vi "Pressure Regulator Test Interface.vi"() -> ()   [LabVIEW 2012, in "Pressure Regulator Controller.lvlib"]
uses:
  Pressure Regulator Controller.lvlib
  <vilib>/express/express shared/transition.llb/Dynamic To Waveform Array.vi
  <vilib>/express/express signal manip/GetorSetDDTAttributes/Shared VIs/XDimension conversion.vi
  <vilib>/express/express signal manip/GetorSetDDTAttributes/Get DDT Attributes/Get DDT Properties.xnode
  <vilib>/express/express signal manip/GetorSetDDTAttributes/Shared VIs/XDimension.ctl
  <vilib>/express/express signal manip/GetorSetDDTAttributes/Shared VIs/GetSetShared.lvlib
panel:
  out "Pressure":dynamicdata(graph)
  out "Signals":dynamicdata(graph)
  in  "stop (F)":bool
  out "error out":errorcluster
  in  "High Level Controls":T1={"Record Button"=FALSE, "Exit"=FALSE, "Hunt"=FALSE, "Break In"=FALSE, "Seal"=FALSE, "Drive In"=FALSE, "Load Pipette"=FALSE, "REC"=FALSE, "File Path Control"=path "D:/Rita Logfiles", "Auto Button"=FALSE, "Auto"=FALSE, "Engage Target"=FALSE, "Abort"=FALSE}
  in  "Calibration Parameters":T2={"Test Signal"={"Seal"={"Amplitude [mV]"=30, "Frequency [hz]"=100}, "Extracellular"={"Amplitude [mV]"=10, "Frequency [hz]"=100}}, "Capacitance Compensation"={"Iterations"=2, "Timeout [ms]"=3000}, "Holding Potential Dynamics"={"Start [mV]"=-70.0, "Target [mV]"=-70.0, "Speed [mV/s]"=0.0}, "Manipulator Dynamics"={"Step length [um]"=2.0, "Interstep Interval [ms]"=3000, "Initial Speed [um/s]"=10.0, "Max Speed [um/s]"=10.0, "Acceleration [um/s^2]"=10.0, "Max Depth [um]"=1200.0, "Max Penetration [um]"=1200.0}, "Suction Parameters"={"Initial Pressure [Kpa]"=0.0, "Minimum Pressure [KPa]"=-40.0, "Decremental Step [KPa]"=-2.0, "Decremental Threshold [%]"=10.0, "Falloff Threshold [%]"=5.0, "Falloff Lag [ms]"=10000.0, "Monitor Refresh [ms]"=3000.0}, "Pressure SPs [KPa]"={"High"=50.0, "Low"=15.0}, "Seal Parameters"={"Seal Target [MOhm]"=1000.0, "Stability Threhsold [%]"=10.0, "Seal Timeout [s]"=600.0, "Stability Refresh [ms]"=3000.0}, "Break in pulse Dynamics"={"Length [ms]"=200.0, "Voltage [mV]"=1000.0, "Pressure [KPa]"=-20.0}, "Unblockage Parameters"={"Blockage Threshold [%]"=5.0, "Max Attempt"=3}, "Targeter Settings"={"Approaching Calibration"={"Approach Factor [um]"=0.9, "Final Clearance [um]"=2.0}, "Optic Flow Settings"={"Pyramid Levels"=6, "Max Iterations"=8, "Displacement Threshold"=0.0, "Window Size"=45}, "Focus"={"Timeout [ms]"=5000, "Max Attempts"=2, "Method"=enum."Continuous"}}} {"Test Signal"."Extracellular"."Frequency [hz]" items=["2 hz "=2, "5 hz"=5, "10 hz "=10, "20 hz"=20, "50 hz"=50, "60 hz"=60, "100 hz"=100, "200 hz"=200, "500 hz"=500, "1000 hz"=1000]; "Test Signal"."Seal"."Frequency [hz]" items=["2 hz "=2, "5 hz"=5, "10 hz "=10, "20 hz"=20, "50 hz"=50, "60 hz"=60, "100 hz"=100, "200 hz"=200, "500 hz"=500, "1000 hz"=1000]}
  in  "Pressure Controls":T3 {"Pressure Sp Manual [KPa]" scale=-50.0..100.0}
  in  "Hardware Configuration":T4={"Pressure Controller Dynamics"={"Positive Branch"={"Kp"=0.0007, "Ki"=0.06, "Kd"=1.0}, "Negative Branch"={"Kp"=0.005, "Ki"=0.005, "Kd"=2.0}}, "Amplifier"={"Multiclamp Serial Number"="00832548", "Multiclamp Channel"=0}, "Manipulator Port"="COM10", "Objective"=600, "Sciscan core Ref"=path "C:/Users/Southampton/Desktop/LUCA_SciScan_141211/GFG/GFG_core.ref", "Signals Sampling"={"Sample Mode"=10123, "Sampling frequecy [hz]"=20000.0, "Samples Number"=1000}, "Electrode Signal"={"Scale Type"=10348, "Terminal Configuration"=10083, "Scale Name"="", "Range [V]"={"max"=10.0, "min"=-10.0}, "Physical Channel"="Dev4/ai2"}, "Pressure Signal"={"Scale Type"=10065, "Terminal Configuration"=10083, "Scale Name"="Compund Pressure", "Range [V]"={"max"=4.0, "min"=0.0}, "Physical Channel"="Dev4/ai4"}, "IIR Filter Specifications"={"Topology"=enum."Off", "Type"=enum."Lowpass", "Order"=0, "Lower Fc"=0.0, "Upper Fc"=0.0, "PB Ripple"=0.0, "SB Attenuation"=0.0}, "Pressure Controller Port"="COM8", "Scope Dynamics"={"Initial Speed [um/s]"=500.0, "Max Speed [um/s]"=1000.0, "Acceleration [um/s^2]"=25.0, "Max Depth [um]"=5000.0}} {"Pressure Signal"."Terminal Configuration" items=["Default"=-1, "RSE"=10083, "Differential"=10106, "Pseudodifferential"=12529]; "Pressure Signal"."Scale Type" items=["Volts"=10348, "Custom Scale"=10065]; "Electrode Signal"."Terminal Configuration" items=["Default"=-1, "RSE"=10083, "Differential"=10106, "Pseudodifferential"=12529]; "Electrode Signal"."Scale Type" items=["Volts"=10348, "Custom Scale"=10065]; "Signals Sampling"."Sample Mode" items=["Finite Samples"=10178, "Continuous Samples"=10123, "Hardware Timed Single Point"=12522]; "Objective" items=["Nikon 16x / 0.80w"=600]; "Amplifier"."Multiclamp Channel" items=["Channel 1", "Channel 2"]}
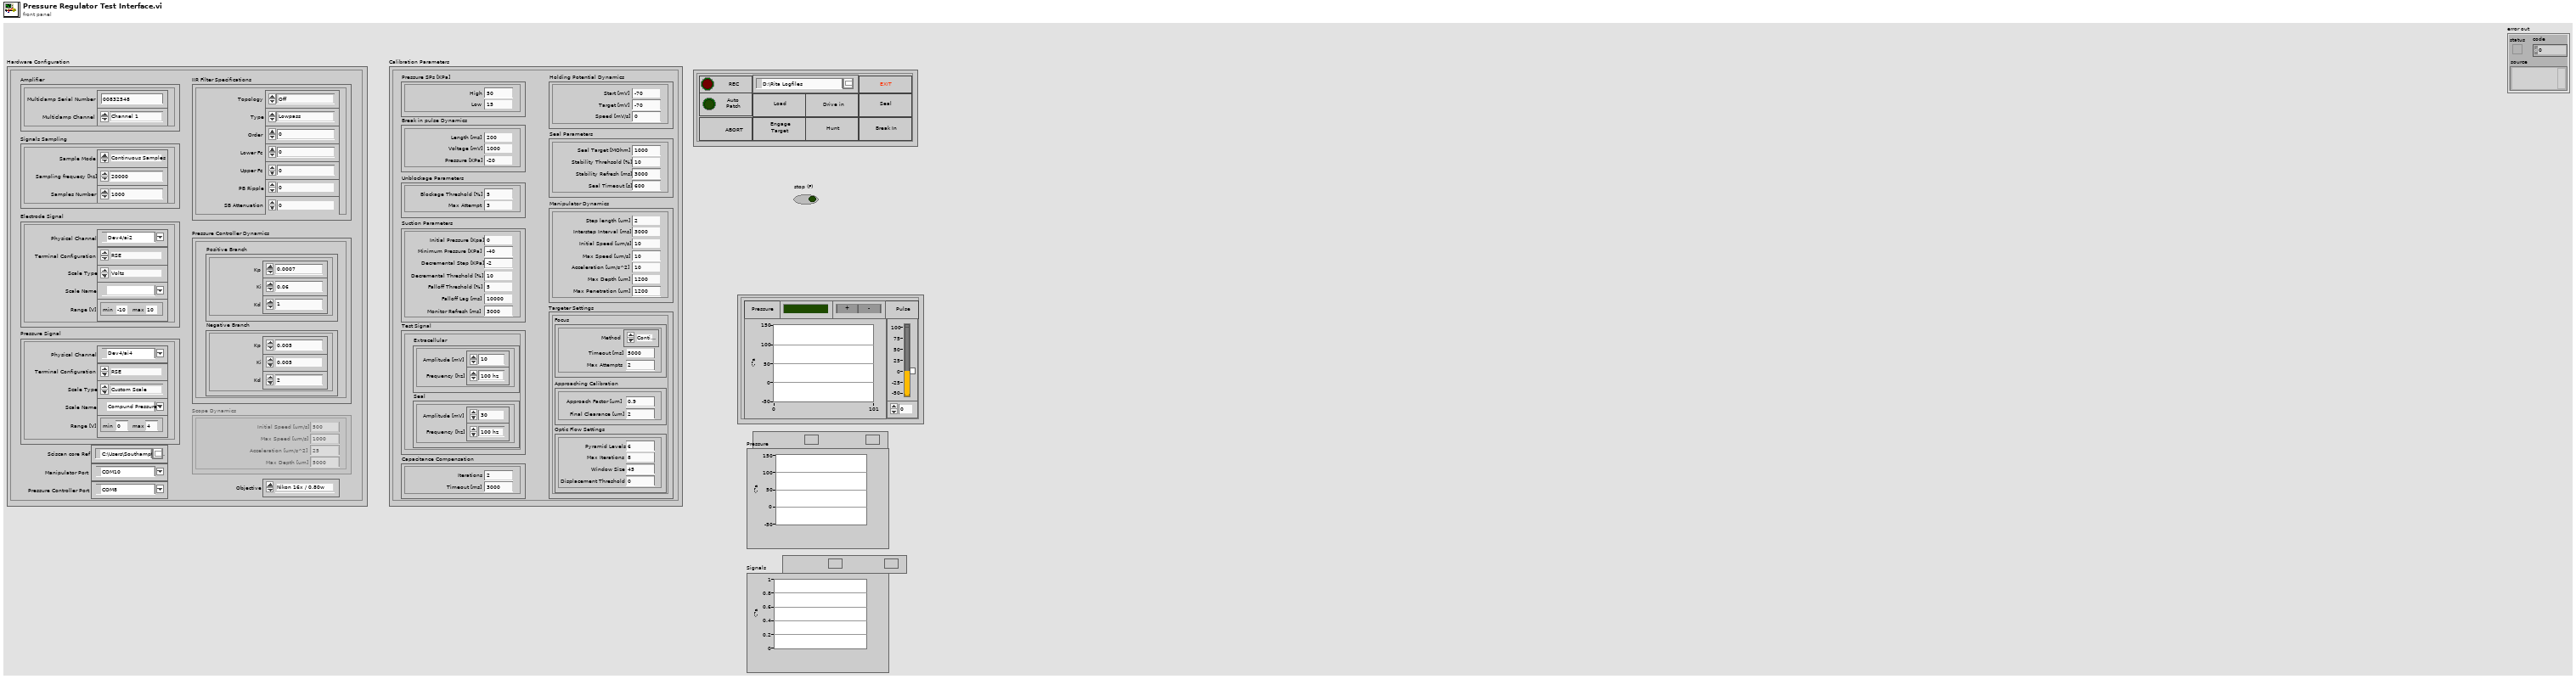
[diagram p1: front panel]
types:
  T1 = cluster{"Record Button":bool, "Exit":bool, "Hunt":bool, "Break In":bool, "Seal":bool, "Drive In":bool, "Load Pipette":bool, "REC":bool, "File Path Control":path, "Auto Button":bool, "Auto":bool, "Engage Target":bool, "Abort":bool}
  T2 = cluster{"Test Signal":cluster{"Seal":cluster{"Amplitude [mV]":i32, "Frequency [hz]":u16}, "Extracellular":cluster{"Amplitude [mV]":i32, "Frequency [hz]":u16}}, "Capacitance Compensation":cluster{"Iterations":i32, "Timeout [ms]":u32}, "Holding Potential Dynamics":cluster{"Start [mV]":dbl, "Target [mV]":dbl, "Speed [mV/s]":dbl}, "Manipulator Dynamics":cluster{"Step length [um]":dbl, "Interstep Interval [ms]":u32, "Initial Speed [um/s]":dbl, "Max Speed [um/s]":dbl, "Acceleration [um/s^2]":dbl, "Max Depth [um]":dbl, "Max Penetration [um]":dbl}, "Suction Parameters":cluster{"Initial Pressure [Kpa]":dbl, "Minimum Pressure [KPa]":dbl, "Decremental Step [KPa]":dbl, "Decremental Threshold [%]":dbl, "Falloff Threshold [%]":dbl, "Falloff Lag [ms]":dbl, "Monitor Refresh [ms]":dbl}, "Pressure SPs [KPa]":cluster{"High":dbl, "Low":dbl}, "Seal Parameters":cluster{"Seal Target [MOhm]":dbl, "Stability Threhsold [%]":dbl, "Seal Timeout [s]":dbl, "Stability Refresh [ms]":dbl}, "Break in pulse Dynamics":cluster{"Length [ms]":dbl, "Voltage [mV]":dbl, "Pressure [KPa]":dbl}, "Unblockage Parameters":cluster{"Blockage Threshold [%]":dbl, "Max Attempt":i32}, "Targeter Settings":cluster{"Approaching Calibration":cluster{"Approach Factor [um]":dbl, "Final Clearance [um]":dbl}, "Optic Flow Settings":cluster{"Pyramid Levels":i32, "Max Iterations":i32, "Displacement Threshold":dbl, "Window Size":i32}, "Focus":cluster{"Timeout [ms]":u32, "Max Attempts":u32, "Method":enum16{"Continuous", "On Demand"}}}}
  T3 = cluster{"Activate Pressure":bool, "Pulse":bool, "Indicator 16":cluster{"Valves":bool}, "Indicator 17":cluster{"Positive Branch":bool, "Negative Branch":bool}, "Pressure Sp Manual [KPa]":dbl, "Pressure Signal":dbl}
  T4 = cluster{"Pressure Controller Dynamics":cluster{"Positive Branch":cluster{"Kp":dbl, "Ki":dbl, "Kd":dbl}, "Negative Branch":cluster{"Kp":dbl, "Ki":dbl, "Kd":dbl}}, "Amplifier":cluster{"Multiclamp Serial Number":string, "Multiclamp Channel":u16}, "Manipulator Port":refnum<visa-resource-name>, "Objective":i16, "Sciscan core Ref":path, "Signals Sampling":cluster{"Sample Mode":i32, "Sampling frequecy [hz]":dbl, "Samples Number":i32}, "Electrode Signal":cluster{"Scale Type":i32, "Terminal Configuration":i32, "Scale Name":tag, "Range [V]":cluster{"max":dbl, "min":dbl}, "Physical Channel":tag}, "Pressure Signal":cluster{"Scale Type":i32, "Terminal Configuration":i32, "Scale Name":tag, "Range [V]":cluster{"max":dbl, "min":dbl}, "Physical Channel":tag}, "IIR Filter Specifications":cluster{"Topology":enum16{"Off", "Butterworth", "Chebyshev", "Inverse Chebyshev", "Elliptic", "Bessel"}, "Type":enum16{"Lowpass", "Highpass", "Bandpass", "Bandstop"}, "Order":i32, "Lower Fc":dbl, "Upper Fc":dbl, "PB Ripple":dbl, "SB Attenuation":dbl}, "Pressure Controller Port":refnum<visa-resource-name>, "Scope Dynamics":cluster{"Initial Speed [um/s]":dbl, "Max Speed [um/s]":dbl, "Acceleration [um/s^2]":dbl, "Max Depth [um]":dbl}}
  T5 = cluster{"Pulse Dynamics":cluster{"Length [ms]":refnum<vi>, "Pressure [KPa] Closed Loop":refnum<vi>, "Voltage [mV] Open Loop":refnum<vi>}, "On/Off":refnum<vi>, "Exit":refnum<vi>, "Pulse":refnum<vi>, "Pressure Sp [KPa]":refnum<vi>, "Pressure Controller Dynamics":refnum<vi>}
  T6 = cluster{"Valves":refnum<vi>, "Branch +":refnum<vi>, "Branch -":refnum<vi>}
  T7 = cluster{"Length [ms]":refnum<vi>, "Pressure [KPa] Closed Loop":refnum<vi>, "Voltage [mV] Open Loop":refnum<vi>}
  T8 = typedef "GetSetShared.lvlib/XDimension.ctl" = enum16{"No Unit [-]", "Time [sec]", "Frequency [Hz]"}
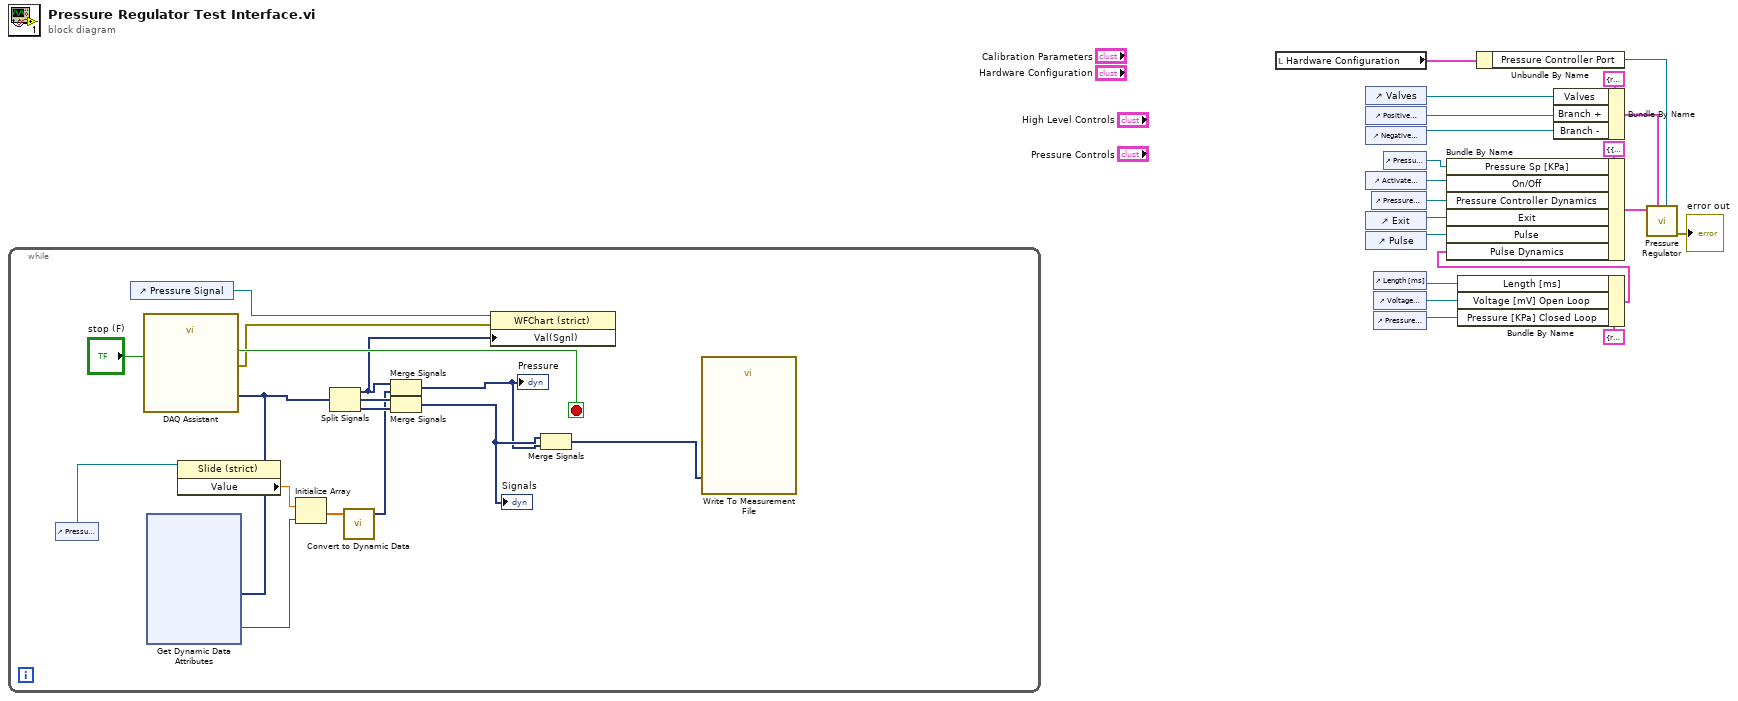
[diagram p0: block diagram]
diagram:
  n1 = while {
    stop <- w35 stop-if-true
    n2 = control-ref of="Pressure Sp Manual [KPa]"() -> (w30:refnum<vi>)
    n3 = control-ref of="Pressure Signal"() -> (w34:refnum<vi>)
    n4 = call "DAQ Assistant"("stop (F)"="stop (F)") -> ("data"=w22:dynamicdata, "stopped"=w35:bool, "error out"=w33:errorcluster)  [unwired: 15 in, 1 out]
    n5 = xnode "Get Dynamic Data Attributes"("Signals In"=w22) -> ("X Dimension"=w21:T8)  [unwired: 2 in, 2 out]
    n6 = property class="Slide (strict)"(reference=w30) -> ("Value"=w28:dbl)  [unwired: 1 in, 2 out]
    n7 = Initialize Array(w28, w21) -> (w27:dbl[])
    n8 = Split Signals(w22) -> (w23:dynamicdata, w32:dynamicdata, w31:dynamicdata)  [unwired: 3 in]
    n9 = call "Convert to Dynamic Data"("Array"=w27) -> ("Dynamic Data Type"=w24:dynamicdata)  [unwired: 3 in]
    n10 = Merge Signals(w23, w24) -> (w25:dynamicdata)
    "Pressure" <- w25
    n11 = Merge Signals(w32, w31) -> (w26:dynamicdata)
    "Signals" <- w26
    n12 = property class="WFChart (strict)"(reference=w34, error in=w33, "Val(Sgnl)"=w23) -> ()  [unwired: 2 out]
    n13 = Merge Signals(w26, w25) -> (w29:dynamicdata)
    n14 = call "Write To Measurement File"("Signals"=w29) -> ()  [unwired: 16 in, 3 out]
  }
  n15 = local read "Hardware Configuration"() -> (w18:T4)
  n16 = control-ref of="Valves"() -> (w12:refnum<vi>)
  n17 = control-ref of="Positive Branch"() -> (w10:refnum<vi>)
  n18 = control-ref of="Negative Branch"() -> (w11:refnum<vi>)
  n19 = control-ref of="Activate Pressure"() -> (w13:refnum<vi>)
  n20 = control-ref of="Exit"() -> (w8:refnum<vi>)
  n21 = control-ref of="Pulse"() -> (w14:refnum<vi>)
  n22 = control-ref of="Pressure Controller Dynamics"() -> (w17:refnum<vi>)
  n23 = control-ref of="Length [ms]"() -> (w4:refnum<vi>)
  n24 = control-ref of="Voltage [mV]"() -> (w6:refnum<vi>)
  n25 = control-ref of="Pressure [KPa]"() -> (w5:refnum<vi>)
  n26 = control-ref of="Pressure Sp Manual [KPa]"() -> (w15:refnum<vi>)
  n27 = Bundle By Name(cluster=T7 {"Length [ms]"=refnum, "Pressure [KPa] Closed Loop"=refnum, "Voltage [mV] Open Loop"=refnum} ("Pulse Dynamics"), "Length [ms]"=w4, "Voltage [mV] Open Loop"=w6, "Pressure [KPa] Closed Loop"=w5) -> (w3:T7)
  n28 = Bundle By Name(cluster=T5 {"Pulse Dynamics"={"Length [ms]"=refnum, "Pressure [KPa] Closed Loop"=refnum, "Voltage [mV] Open Loop"=refnum}, "On/Off"=refnum, "Exit"=refnum, "Pulse"=refnum, "Pressure Sp [KPa]"=refnum, "Pressure Controller Dynamics"=refnum} ("Controls"), "Pressure Sp [KPa]"=w15, "On/Off"=w13, "Pressure Controller Dynamics"=w17, "Exit"=w8, "Pulse"=w14, "Pulse Dynamics"=w3) -> (w19:T5)
  n29 = Unbundle By Name(w18) -> ("Pressure Controller Port"=w20:refnum<visa-resource-name>)
  n30 = Bundle By Name(cluster=T6 {"Valves"=refnum, "Branch +"=refnum, "Branch -"=refnum} ("Indicators"), "Valves"=w12, "Branch +"=w10, "Branch -"=w11) -> (w9:T6)
  n31 = call "Pressure Regulator.vi"("Indicators"=w9, "Pressure Controller Port"=w20, "Controls"=w19) -> ("error out"=→"error out":errorcluster)  [unwired: 8 in]
